vi "Parse Python Message.vi"(8 "error in":errorcluster, 10 "Python Message":string) -> (0 "error out":errorcluster, 1 "Argument String":string, 2 "PYTHON Command":string, 3 "PYTHON Node Name":string)   [LabVIEW 2020, in "jki_python_bridge.lvlib" / "Server.lvclass"]
uses:
  Server.lvclass
  <userlib>/_OpenG.lib/string/string.llb/Trim Whitespace (String)__ogtk.vi
  <userlib>/_OpenG.lib/string/string.llb/openg_string.lvlib
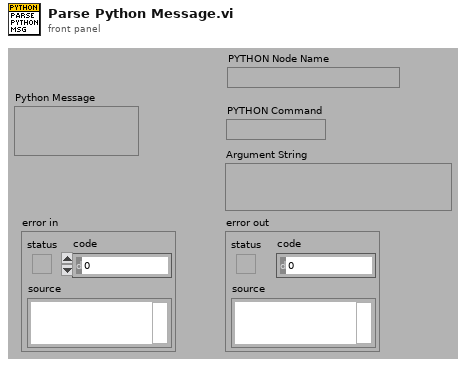
[diagram p1: front panel]
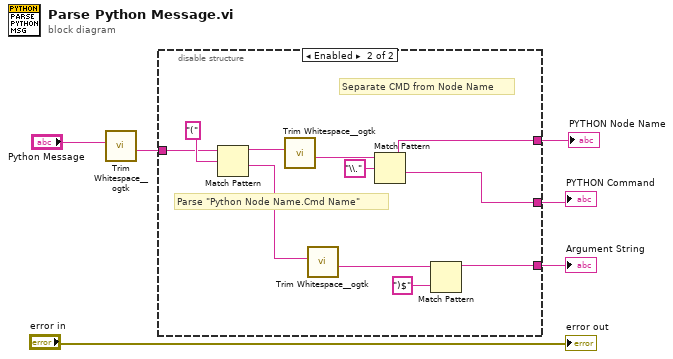
[diagram p0: block diagram]
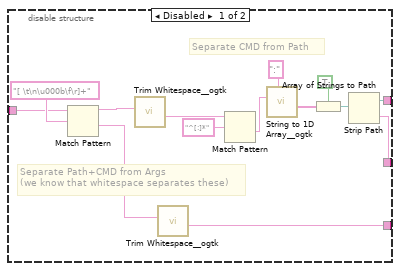
[diagram p2: hidden frame]
diagram:
  n1 = call-poly <userlib>:"Trim Whitespace__ogtk.vi"("String in"="Python Message") -> ("String out"=w6:string)  [unwired: 6 in]
  n2 = disable-structure shown="Enabled" {
    disable-tunnel: w6 -> [w19 w30]
    disable-tunnel: [w17 w21] -> w3
    disable-tunnel: [w13 w25] -> w5
    disable-tunnel: [w12 w24] -> w4
    frame Disabled {
      # "Separate CMD from Path"
      # "Separate Path+CMD from Args\n(we know that whitespace separates these)"
      n3 = Match Pattern(string=w19, regular expression="[ \t\n\u000b\f\r]+") -> (before substring=w16:string, after substring=w18:string)  [unwired: 1 in, 2 out]
      n4 = call-poly <userlib>:"Trim Whitespace__ogtk.vi"("String in"=w16) -> ("String out"=w10:string)  [unwired: 6 in]
      n5 = call-poly <userlib>:"Trim Whitespace__ogtk.vi"("String in"=w18) -> ("String out"=w17:string)  [unwired: 6 in]
      n6 = Match Pattern(string=w10, regular expression="^[:]*") -> (after substring=w8:string)  [unwired: 1 in, 3 out]
      n7 = call <userlib>:"String to 1D Array__ogtk.vi"("delimiter (Tab)"=":", "string"=w8) -> ("Array of Strings"=w7:string[])  [unwired: 9 in]
      n8 = Array of Strings to Path(0:w7, 1:TRUE ("relative")) -> (2:w14:path)
      n9 = Strip Path(path=w14) -> (stripped path=w13:path, name=w12:string)
    }
    frame Enabled {
      # "Separate CMD from Node Name"
      # "Parse \"Python Node Name.Cmd Name\""
      n10 = Match Pattern(string=w30, regular expression="(") -> (before substring=w28:string, after substring=w29:string)  [unwired: 1 in, 2 out]
      n11 = call-poly <userlib>:"Trim Whitespace__ogtk.vi"("String in"=w28) -> ("String out"=w27:string)  [unwired: 6 in]
      n12 = call-poly <userlib>:"Trim Whitespace__ogtk.vi"("String in"=w29) -> ("String out"=w22:string)  [unwired: 6 in]
      n13 = Match Pattern(string=w27, regular expression="\\.") -> (before substring=w25:string, after substring=w24:string)  [unwired: 1 in, 2 out]
      n14 = Match Pattern(string=w22, regular expression=")$") -> (before substring=w21:string)  [unwired: 1 in, 3 out]
    }
  }
  "PYTHON Command" <- w4
  "Argument String" <- w3
  "PYTHON Node Name" <- w5
  "error out" <- "error in"
